vi "Write sort_.vi"(8 "error in":errorcluster, 10 "sort?":bool, 11 "user tag bus module editor node in":refnum<class "TEST EDITOR.lvclass">) -> (0 "error out":errorcluster, 3 "user tag bus module editor node out":refnum<class "TEST EDITOR.lvclass">)   [LabVIEW 2013, in "configuration tests.lvlib" / "TEST EDITOR.lvclass"]
uses:
  TEST EDITOR.lvclass
  TEST EDITOR.lvclass/TEST EDITOR.ctl
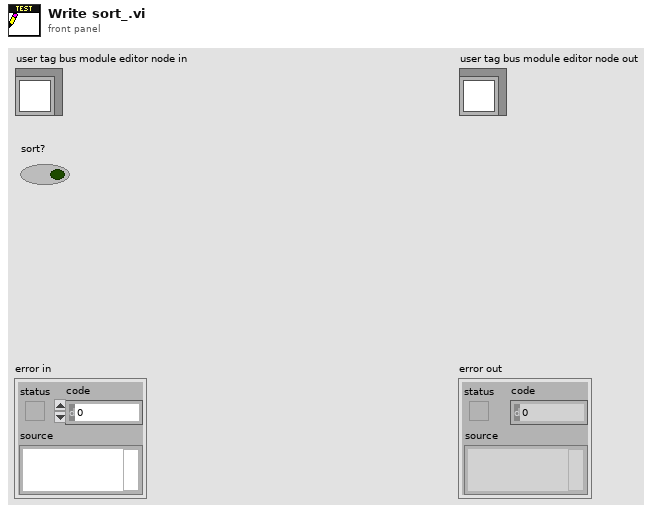
[diagram p1: front panel]
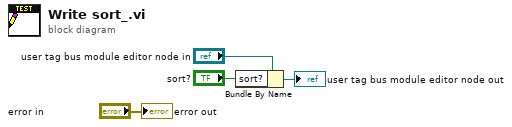
[diagram p0: block diagram]
diagram:
  n1 = Bundle By Name(cluster="user tag bus module editor node in", "sort?"="sort?") -> (→"user tag bus module editor node out":refnum<class "TEST EDITOR.lvclass">)
  "error out" <- "error in"
